vi "WPI_PWMDoesDevRefExist.vi"(0 "PWMDeviceRefArray":T1[](array[typedef]), 7 "PWMDeviceRef":T1={"DeviceStatus"={"status"=FALSE, "code"=0, "source"=""}, "PWM Channel"=enum."PWM 1"}) -> (4 "index":i32, 8 "exists":bool)   [LabVIEW 2017]
doc: "This is used to find the index of a DevRef within an array of DevRefs."
uses:
  <vilib>/Rock Robotics/WPI/PWM/WPI_PWMDeviceRef.ctl
  <vilib>/Rock Robotics/SystemInterfaces/DIO/FPGA_DIOPWMChannel.ctl
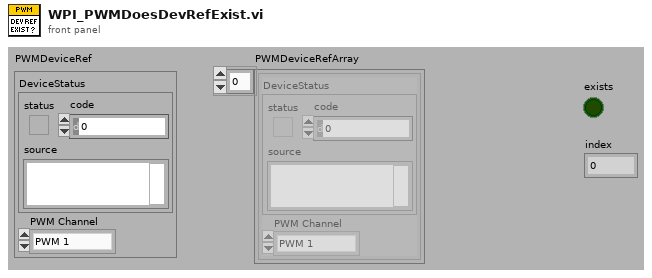
[diagram p1: front panel]
types:
  T1 = typedef "WPI_PWMDeviceRef.ctl" = cluster{"DeviceStatus":errorcluster, "PWM Channel":T2}
  T2 = typedef "FPGA_DIOPWMChannel.ctl" = enum8{"PWM 0", "PWM 1", "PWM 2", "PWM 3", "PWM 4", "PWM 5", "PWM 6", "PWM 7", "PWM 8", "PWM 9", "PWM MXP 0", "PWM MXP 1", "PWM MXP 2", "PWM MXP 3", "PWM MXP 4", "PWM MXP 5", "PWM MXP 6", "PWM MXP 7", "PWM MXP 8", "PWM MXP 9", "Invalid"}
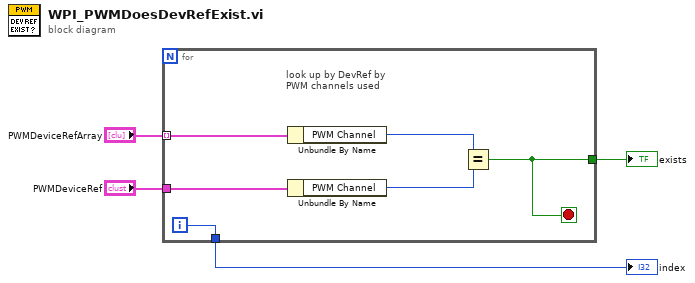
[diagram p0: block diagram]
diagram:
  n1 = for {
    tunnel: "PWMDeviceRefArray" -> [w10] mode=indexing
    tunnel: "PWMDeviceRef" -> [w9]
    tunnel: [w8] -> w2
    tunnel: [w7] -> w1
    i -> [w7]
    stop <- w8 stop-if-true
    # "look up by DevRef by PWM channels used"
    n2 = Unbundle By Name(w10) -> ("PWM Channel"=w6:T2)
    n3 = Unbundle By Name(w9) -> ("PWM Channel"=w5:T2)
    n4 = Equal?(x=w6, y=w5) -> (x = y?=w8:bool)
  }
  "exists" <- w2
  "index" <- w1
